vi "Duplicate Name Error Test.vi"() -> (0 "error out":errorcluster, 1 "Success Error on Replace Line":bool, 2 "Success Error on Write Lines":bool, 3 "Success Error on Add":bool, 4 "Pass":bool)   [LabVIEW 2021, in "Multiplexer tests.lvlib"]
doc: "Tests the Add Line and Remove Line functions."
uses:
  Multiplexer tests.lvlib
  <vilib>/NI/Tag Bus/tag/Data Type.ctl
  configuration/Line.ctl
  <vilib>/NI/Tag Bus Module Framework/channel/TBM channel.lvclass
  configuration/permissions.ctl
  configuration/Get Line Name.vi
  <vilib>/NI/Tag Bus Module Framework/module configuration/FindDuplicate.vi
  <vilib>/Utility/error.llb/Error Cluster From Error Code.vi
  configuration/Multiplexer configuration.lvclass
  <vilib>/NI/Tag Bus/tag/tag descriptor.lvclass
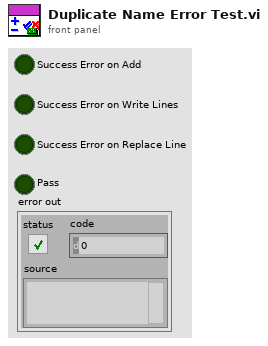
[diagram p1: front panel]
types:
  T1 = typedef "Multiplexer configuration.lvclass/permissions.ctl" = enum32{"Read from HW", "Write to HW"}
  T2 = typedef "Multiplexer configuration.lvclass/Line.ctl" = cluster{"A":refnum<class "TBM channel.lvclass">, "B":refnum<class "TBM channel.lvclass">, "Select":refnum<class "TBM channel.lvclass">, "Output":refnum<class "TBM channel.lvclass">}
  T3 = typedef "tag bus.lvlib/tag descriptor.lvclass/Data Type.ctl" = enum16{"Double", "Single", "I64", "I32", "I16", "I8", "U64", "U32", "U16", "U8", "Boolean", "String", "Array of Double", "Array of Single", "Array of I64", "Array of I32", "Array of I16", "Array of I8", "Array of U64", "Array of U32", "Array of U16", "Array of U8", "Array of Boolean", "Array of String"}
  T4 = typedef "TBM channel.lvclass/channel classification.ctl" = enum16{"input data", "output data", "processing parameter", "processing result"}
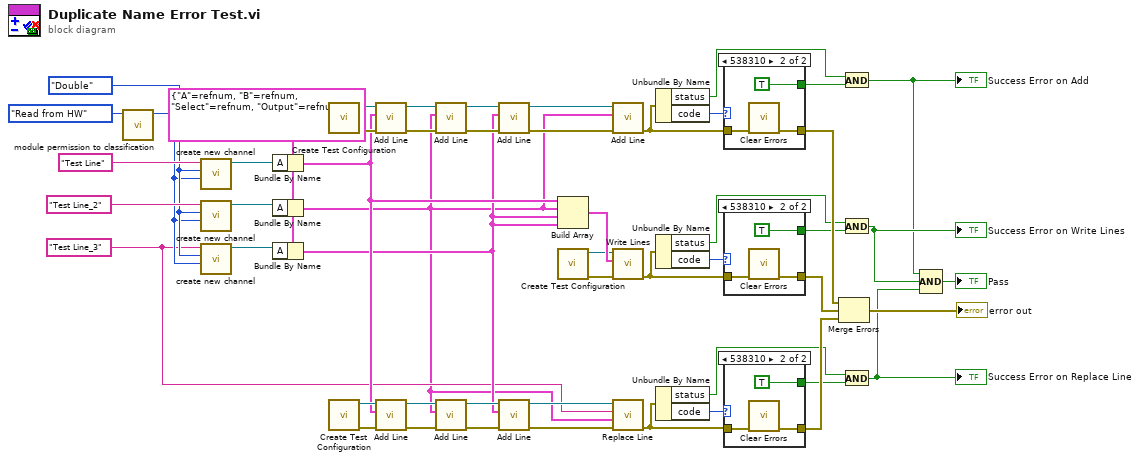
[diagram p0: block diagram]
diagram:
  w17 = "Test Line_3" ("channel name")
  w44 = T2 {"A"=refnum, "B"=refnum, "Select"=refnum, "Output"=refnum} ("Line")
  w39 = Data_Type."Double" ("data type")
  n1 = call "module permission to classification.vi"("display permissions"=permissions."Read from HW") -> ("channel classification"=w38:T4)  [unwired: 10 in]
  n2 = call <vilib>:"create new channel.vi"("channel classification"=w38, "data type"=w39, "channel name"="Test Line") -> ("channel"=w51:refnum<class "TBM channel.lvclass">)  [unwired: 8 in]
  n3 = call <vilib>:"create new channel.vi"("channel classification"=w38, "data type"=w39, "channel name"="Test Line_2") -> ("channel"=w46:refnum<class "TBM channel.lvclass">)  [unwired: 8 in]
  n4 = call <vilib>:"create new channel.vi"("channel classification"=w38, "data type"=w39, "channel name"=w17) -> ("channel"=w45:refnum<class "TBM channel.lvclass">)  [unwired: 8 in]
  n5 = Bundle By Name(cluster=w44, "A"=w51) -> (w20:T2)
  n6 = Bundle By Name(cluster=w44, "A"=w46) -> (w16:T2)
  n7 = Bundle By Name(cluster=w44, "A"=w45) -> (w19:T2)
  n8 = call "Create Test Configuration.vi"() -> ("error out"=w50:errorcluster, "Module Configuration"=w52:refnum<class "Multiplexer configuration.lvclass">)  [unwired: 6 in, 4 out]
  n9 = call "Create Test Configuration.vi"() -> ("error out"=w22:errorcluster, "Module Configuration"=w21:refnum<class "Multiplexer configuration.lvclass">)  [unwired: 6 in, 4 out]
  n10 = call "Add Line.vi"("error in"=w50, "Line"=w20, "Multiplexer configuration in"=w52) -> ("error out"=w43:errorcluster, "Multiplexer configuration out"=w40:refnum<class "Multiplexer configuration.lvclass">)  [unwired: 6 in, 1 out]
  n11 = call "Add Line.vi"("error in"=w22, "Line"=w20, "Multiplexer configuration in"=w21) -> ("error out"=w23:errorcluster, "Multiplexer configuration out"=w26:refnum<class "Multiplexer configuration.lvclass">)  [unwired: 6 in, 1 out]
  n12 = call "Add Line.vi"("error in"=w43, "Line"=w16, "Multiplexer configuration in"=w40) -> ("error out"=w42:errorcluster, "Multiplexer configuration out"=w41:refnum<class "Multiplexer configuration.lvclass">)  [unwired: 6 in, 1 out]
  n13 = call "Add Line.vi"("error in"=w23, "Line"=w16, "Multiplexer configuration in"=w26) -> ("error out"=w24:errorcluster, "Multiplexer configuration out"=w25:refnum<class "Multiplexer configuration.lvclass">)  [unwired: 6 in, 1 out]
  n14 = call "Add Line.vi"("error in"=w42, "Line"=w19, "Multiplexer configuration in"=w41) -> ("error out"=w36:errorcluster, "Multiplexer configuration out"=w37:refnum<class "Multiplexer configuration.lvclass">)  [unwired: 6 in, 1 out]
  n15 = call "Add Line.vi"("error in"=w24, "Line"=w19, "Multiplexer configuration in"=w25) -> ("error out"=w15:errorcluster, "Multiplexer configuration out"=w18:refnum<class "Multiplexer configuration.lvclass">)  [unwired: 6 in, 1 out]
  n16 = Build Array(w20, w16, w19, w19) -> (w33:T2[])
  n17 = call "Create Test Configuration.vi"() -> ("error out"=w14:errorcluster, "Module Configuration"=w32:refnum<class "Multiplexer configuration.lvclass">)  [unwired: 6 in, 4 out]
  n18 = call "Add Line.vi"("error in"=w36, "Line"=w16, "Multiplexer configuration in"=w37) -> ("error out"=w34:errorcluster)  [unwired: 6 in, 2 out]
  n19 = call "Write Lines.vi"("error in (no error)"=w14, "Lines"=w33, "Multiplexer configuration in"=w32) -> ("error out"=w30:errorcluster)  [unwired: 7 in, 1 out]
  n20 = call "Replace Line.vi"("error in"=w15, "New Line"=w16, "Line Name"=w17, "Multiplexer configuration in"=w18) -> ("error out"=w12:errorcluster)  [unwired: 5 in, 2 out]
  n21 = Unbundle By Name(w34) -> ("status"=w9:bool, "code"=w35:i32)
  n22 = Unbundle By Name(w30) -> ("status"=w6:bool, "code"=w31:i32)
  n23 = Unbundle By Name(w12) -> ("status"=w7:bool, "code"=w13:i32)
  n24 = case shown="538310" w35 {
    tunnel: w34 -> [w53 w56]
    tunnel: [w53 w55] -> w29
    tunnel: [_ TRUE ("Success Error on Add")] -> w10
    frame 0, Default {
    }
    frame 538310 {
      n25 = call <vilib>:"Clear Errors.vi"("error in (no error)"=w56) -> ("error out"=w55:errorcluster)  [unwired: 5 in, 1 out]
    }
  }
  n26 = case shown="538310" w31 {
    tunnel: w30 -> [w57 w60]
    tunnel: [w57 w59] -> w28
    tunnel: [_ TRUE ("Success Error on Add")] -> w5
    frame 0, Default {
    }
    frame 538310 {
      n27 = call <vilib>:"Clear Errors.vi"("error in (no error)"=w60) -> ("error out"=w59:errorcluster)  [unwired: 5 in, 1 out]
    }
  }
  n28 = case shown="538310" w13 {
    tunnel: w12 -> [w61 w64]
    tunnel: [w61 w63] -> w11
    tunnel: [_ TRUE ("Success Error on Add")] -> w8
    frame 0, Default {
    }
    frame 538310 {
      n29 = call <vilib>:"Clear Errors.vi"("error in (no error)"=w64) -> ("error out"=w63:errorcluster)  [unwired: 5 in, 1 out]
    }
  }
  n30 = Merge Errors(w29, w28, w11) -> (→"error out":errorcluster)
  n31 = And(x=w9, y=w10) -> (x .and. y?=w2:bool)
  "Success Error on Add" <- w2
  n32 = And(x=w6, y=w5) -> (x .and. y?=w3:bool)
  "Success Error on Write Lines" <- w3
  n33 = And(x=w7, y=w8) -> (x .and. y?=w4:bool)
  "Success Error on Replace Line" <- w4
  n34 = Compound Arithmetic op=AND(w2, w3, w4) -> (→"Pass":bool)
